vi "add or delete location.vi"(6 "Function":u16(ring) items=["Add/set", "Delete"], 7 "List of defaults":T1 {"List of locations"."Position"."Position Y" format="%#.3f"; "List of locations"."Position"."Position X" format="%#.3f"}, 8 "New location":T3 {"Position"."Position Y" format="%#.3f"; "Position"."Position X" format="%#.3f"}, 9 "Location in":u16, 10 "Device in":u16, 11 "List of devices in":T1 {"List of locations"."Position"."Position Y" format="%#.3f"; "List of locations"."Position"."Position X" format="%#.3f"}) -> (1 "Location out":u16, 2 "Device out":u16, 3 "List of devices out":T1 {"List of locations"."Position"."Position Y" format="%#.3f"; "List of locations"."Position"."Position X" format="%#.3f"})   [LabVIEW 2017]
uses:
  device_list.ctl
  device.ctl
  location.ctl
  <vilib>/Utility/miscctls.llb/LVPointTypeDef.ctl
panel:
  in  "Cancel Button 2":bool
  in  "Delete Button":bool
  in  "Location - delete":u16(ring) caption="Location" items=["Center", "<all>"]
  in  "Device - delete":u16(ring) caption="Device" items=["Layout", "<all>"]
  in  "What to shift?":enum32{"Location", "Device", "All devices"}(radio)
  in  "Location description":string
  in  "Device description":string
  in  "OK Button":bool
  in  "Cancel Button":bool
  in  "Location":u16(ring) items=["Center", "<new location>"]
  in  "Device":u16(ring) items=["Layout", "<new device>"]
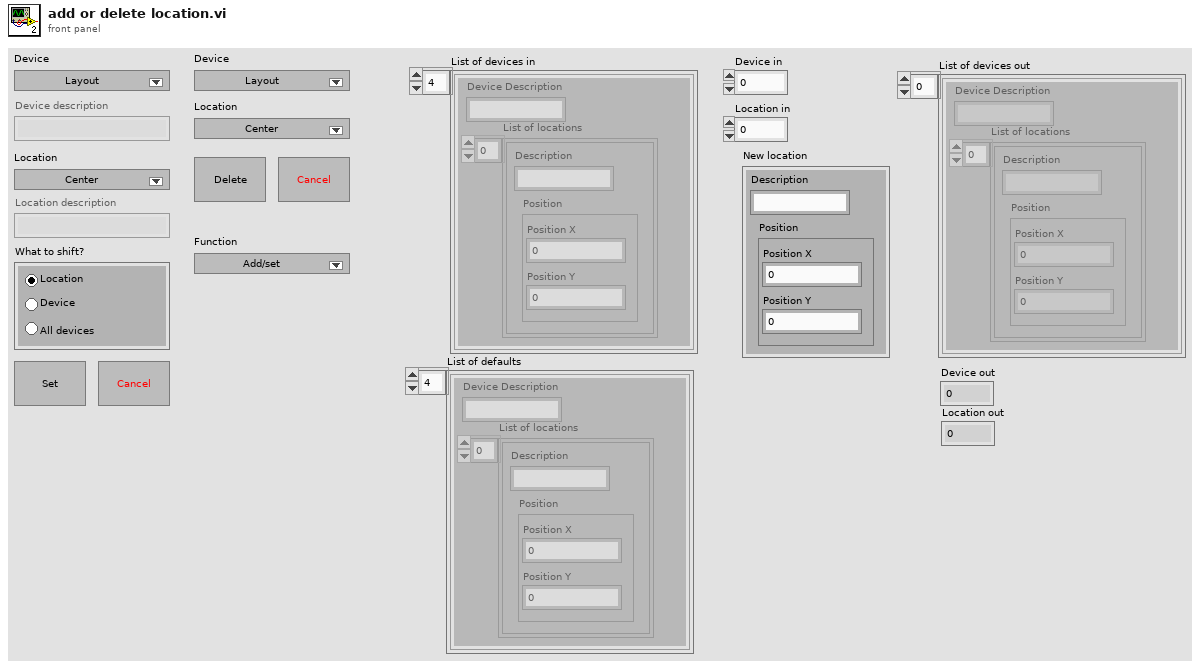
[diagram p1: front panel]
types:
  T1 = typedef "device_list.ctl" = T2[]
  T2 = typedef "device.ctl" = cluster{"List of locations":T3[], "Device Description":string}
  T3 = typedef "location.ctl" = cluster{"Description":string, "Position":cluster{"Position X":dbl, "Position Y":dbl}}
  T4 = typedef "LVRectTypeDef.ctl" = cluster{"Left":i16, "Top":i16, "Right":i16, "Bottom":i16}
  T5 = typedef "LVPointTypeDef.ctl" = cluster{"Horizontal":i16, "Vertical":i16}
  T6 = enum8{"Enabled", "Disabled", "Disabled and Grayed Out"}
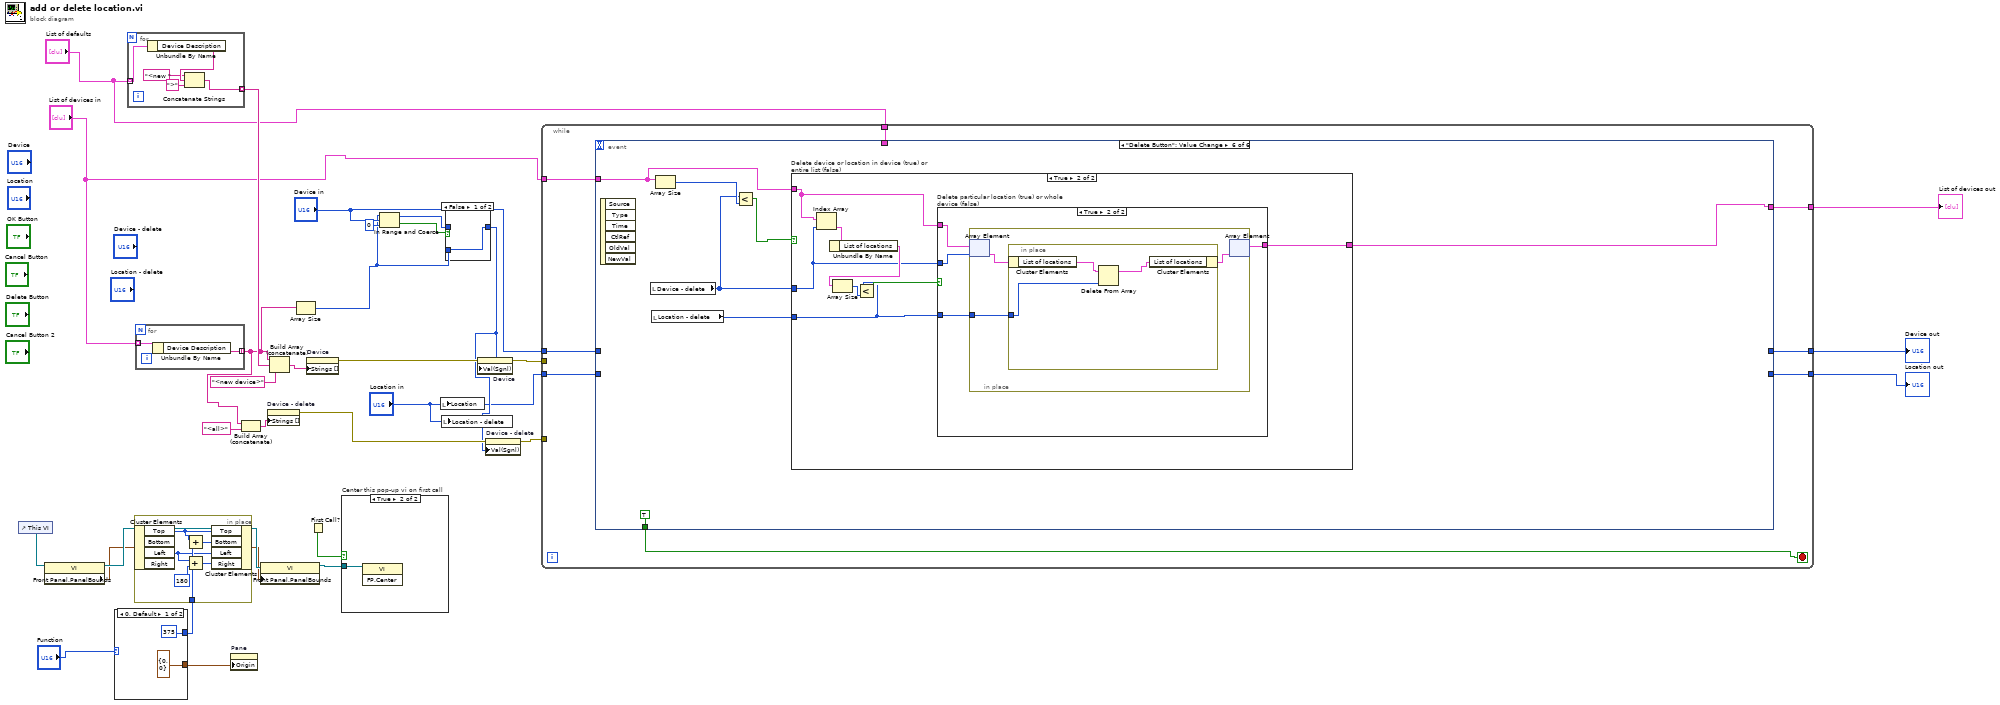
[diagram p0: block diagram]
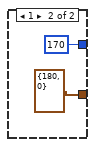
[diagram p2: hidden frame]
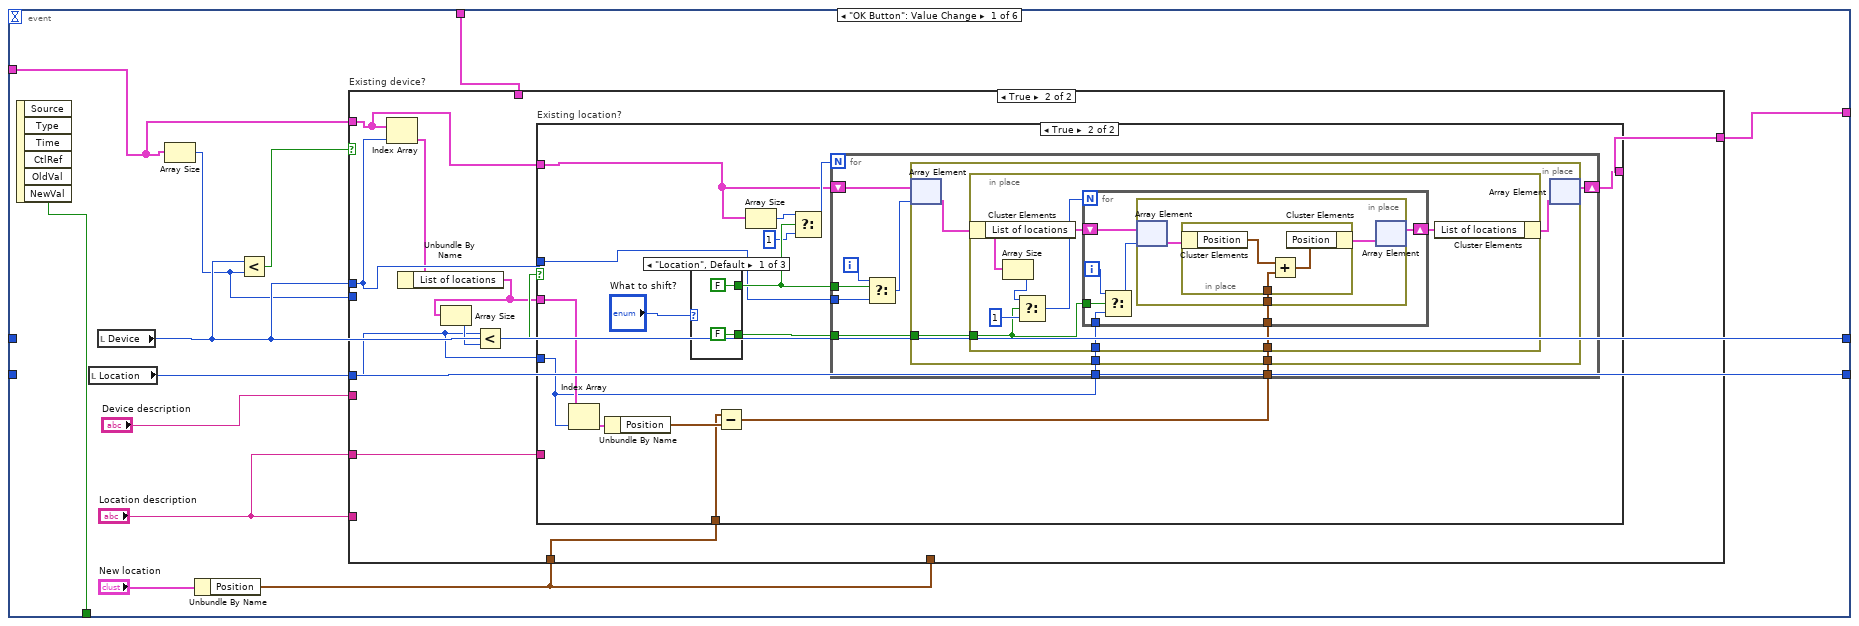
[diagram p5: hidden frame]
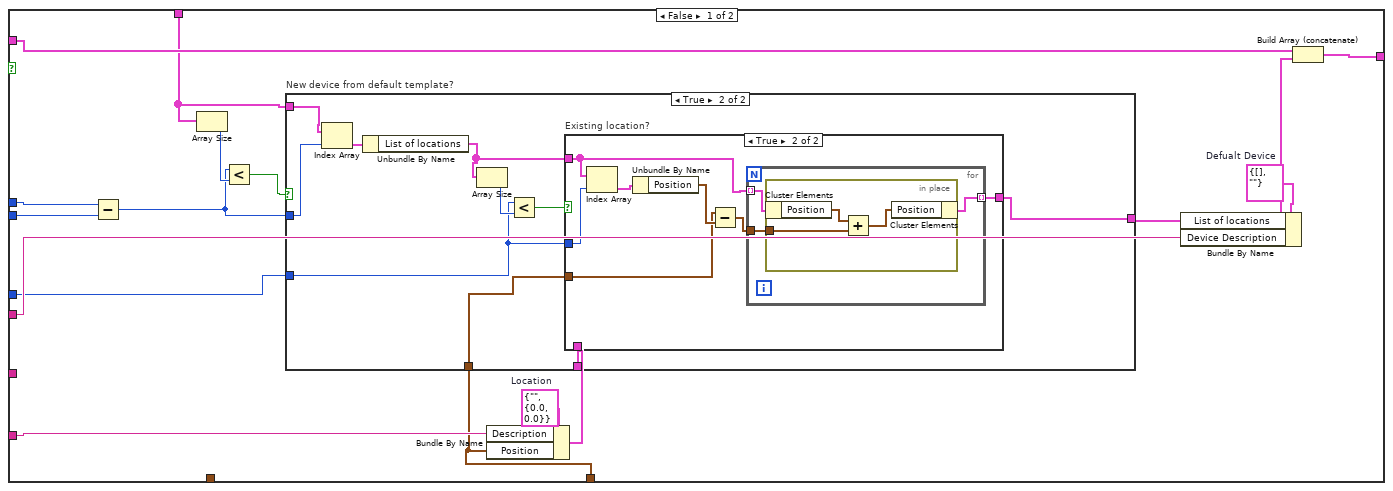
[diagram p6: hidden frame]
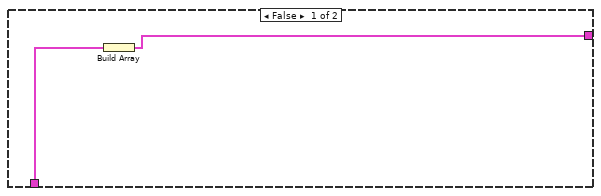
[diagram p7: hidden frame]
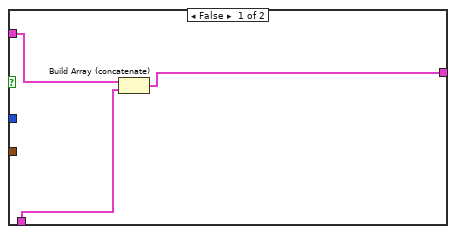
[diagram p8: hidden frame]
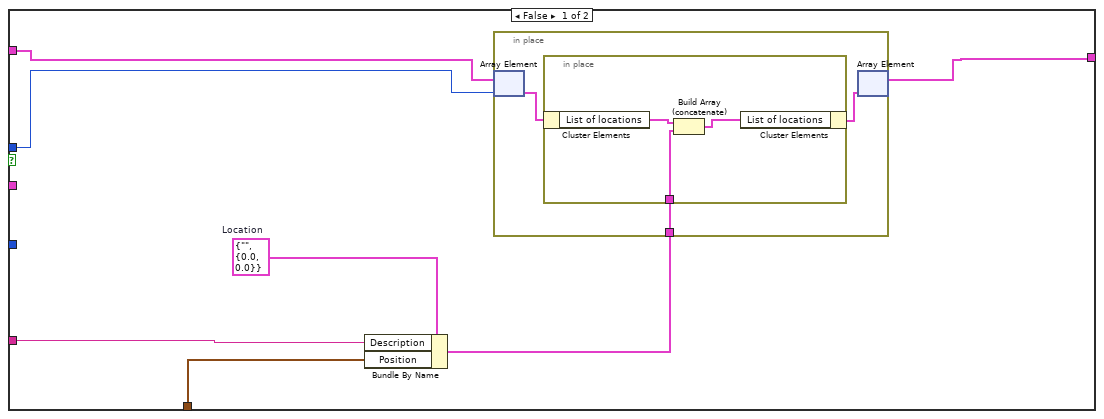
[diagram p9: hidden frame]
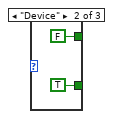
[diagram p10: hidden frame]
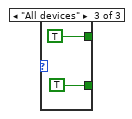
[diagram p11: hidden frame]
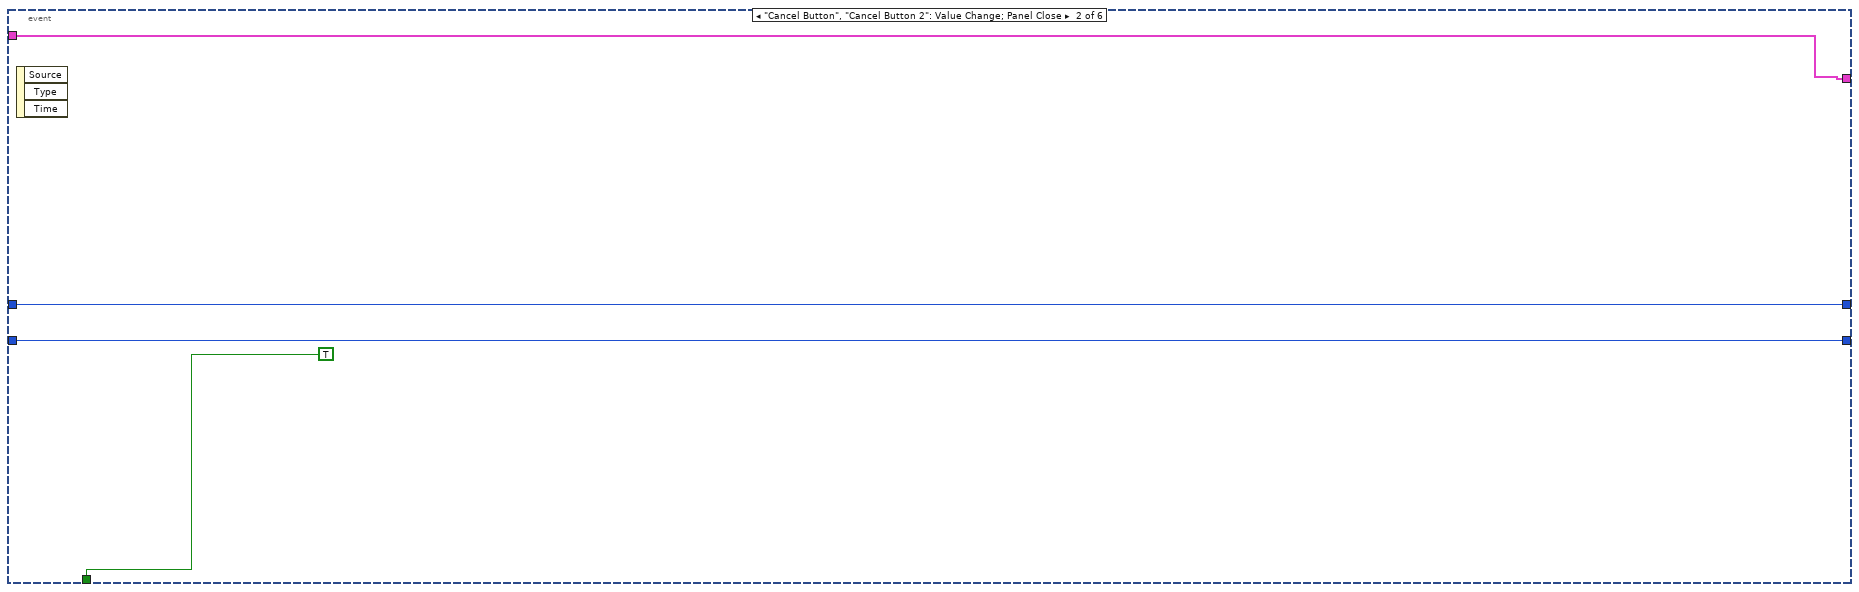
[diagram p12: hidden frame]
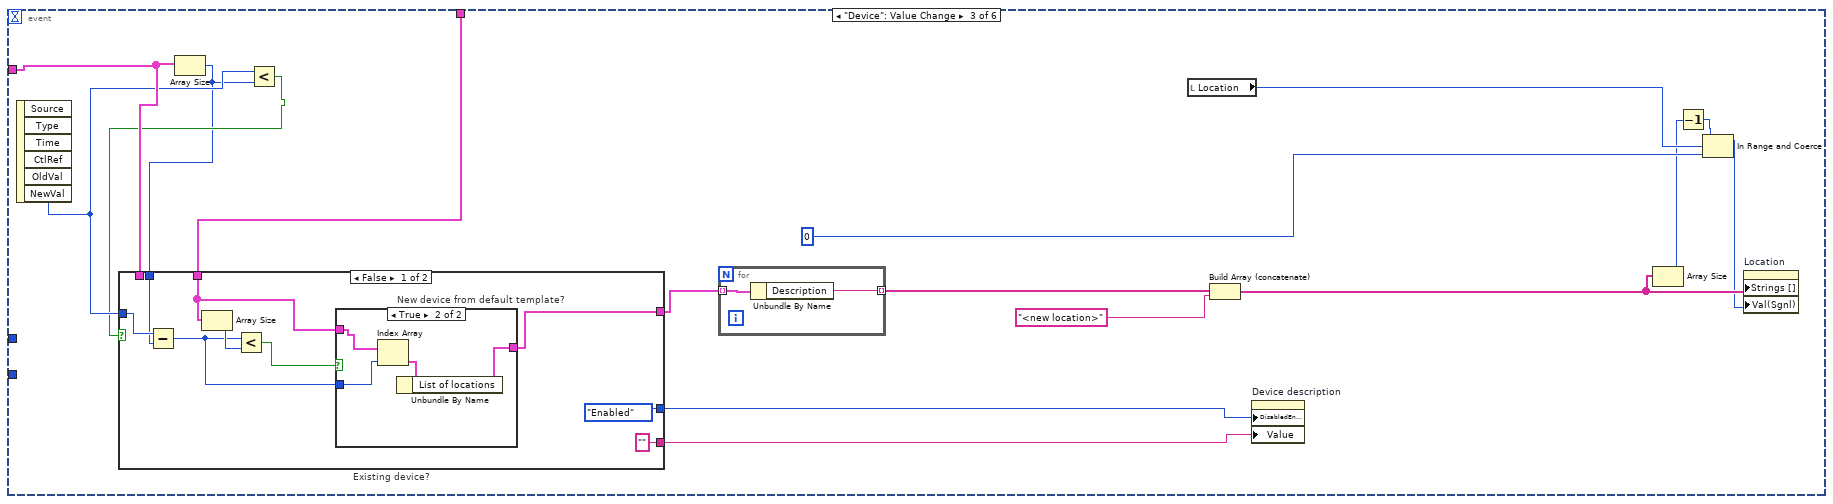
[diagram p13: hidden frame]
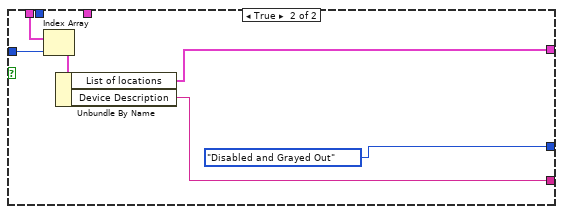
[diagram p15: hidden frame]
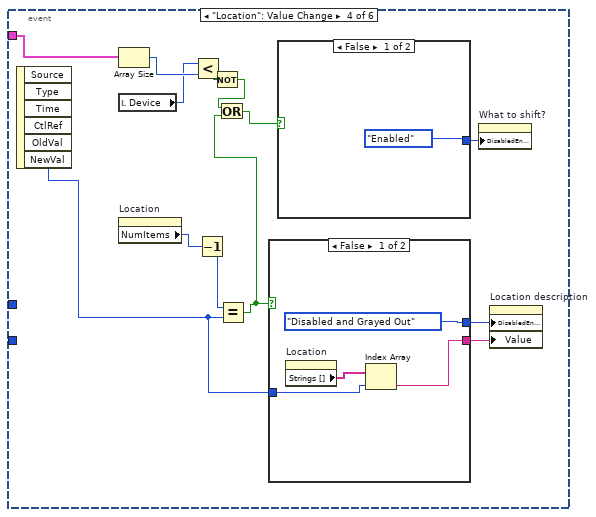
[diagram p16: hidden frame]
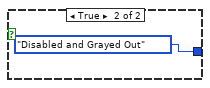
[diagram p17: hidden frame]
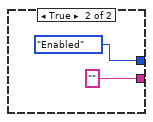
[diagram p18: hidden frame]
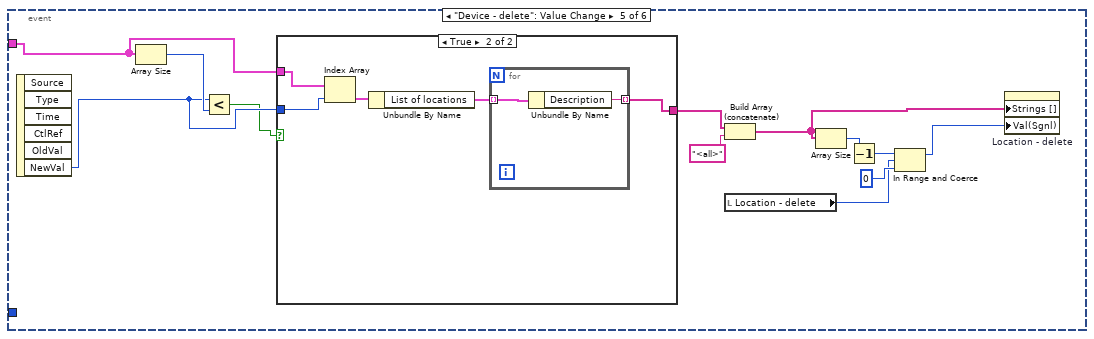
[diagram p19: hidden frame]
diagram:
  n1 = control-ref of="This VI"() -> (w6:refnum<vi>)
  n2 = property class="VI"(reference=w6) -> (reference out=w5:refnum<vi>, "Front Panel.PanelBounds"=w2:T4)  [unwired: 1 in, 1 out]
  n3 = case shown="0, Default" "Function" {
    tunnel: [T5 {"Horizontal"=0, "Vertical"=0} ("Origin") T5 {"Horizontal"=180, "Vertical"=0} ("Origin")] -> w8
    tunnel: [i16 375 ("Horizontal") i16 170 ("Horizontal")] -> w1
    frame 0, Default {
    }
    frame 1 {
    }
  }
  n4 = for {
    tunnel: "List of defaults" -> [w40] mode=indexing
    tunnel: [w36] -> w25 mode=indexing
    n5 = Unbundle By Name(w40) -> ("Device Description"=w39:string)
    n6 = Concatenate Strings("<new " ("string"), w39, ">" ("string")) -> (w36:string)
  }
  n7 = in-place {
    in-place-border: w1 -> [w42]
    n8 = in-place-cluster #1(w2) -> ("Top"=w46:i16, "Left"=w41:i16)  [unwired: 2 out]
    n9 = Add(x=w41, y=i16 180) -> (x+y=w43:i16)
    n10 = Add(x=w46, y=w42) -> (x+y=w45:i16)
    n11 = in-place-cluster #1("Top"=w46, "Bottom"=w45, "Left"=w41, "Right"=w43) -> (w4:T4)
  }
  n12 = for {
    tunnel: "List of devices in" -> [w48] mode=indexing
    tunnel: [w47] -> w19 mode=indexing
    n13 = Unbundle By Name(w48) -> ("Device Description"=w47:string)
  }
  n14 = property on="Pane" class="Pane"("Origin"=w8) -> ()  [unwired: 2 in, 2 out]
  n15 = Build Array (concatenate)(w19, "<all>" ("Device Description")) -> (w17:string[])
  n16 = property class="VI"(reference=w5, "Front Panel.PanelBounds"=w4) -> (reference out=w3:refnum<vi>)  [unwired: 1 in, 1 out]
  n17 = property on="Device - delete" class="Ring (strict)"("Strings []"=w17) -> (error out=w16:errorcluster)  [unwired: 2 in, 1 out]
  n18 = Build Array (concatenate)(w19, w25, "<new device>" ("Device Description")) -> (w24:string[])
  n19 = Array Size(array=w19) -> (size(s)=w13:i32)
  n20 = property on="Device" class="Ring (strict)"("Strings []"=w24) -> (error out=w28:errorcluster)  [unwired: 2 in, 1 out]
  n21 = First Call?() -> (First Call?: T/F=w20:bool)
  n22 = case "Center this pop-up vi on first call" shown="True" w20 {
    tunnel: w3 -> [_ w49]
    frame False {
    }
    frame True {
      n23 = invoke class="VI" method="FP.Center"(reference=w49) -> ()  [unwired: 2 in, 3 out]
    }
  }
  n24 = In Range and Coerce(upper limit=w13, x="Device in", lower limit=0) -> (coerced(x)=w12:i32, In Range?=w11:bool)
  n25 = local write "Location"("Location in") -> ()
  n26 = local write "Location - delete"("Location in") -> ()
  n27 = case shown="False" w11 {
    tunnel: w12 -> [_ w51]
    tunnel: [w50 w51] -> w10
    tunnel: w13 -> [w50 _]
    frame False {
    }
    frame True {
    }
  }
  n28 = property on="Device" class="Ring (strict)"(error in=w28, "Val(Sgnl)"=w10) -> (error out=w27:errorcluster)  [unwired: 1 in, 1 out]
  n29 = property on="Device - delete" class="Ring (strict)"(error in=w16, "Val(Sgnl)"=w10) -> (error out=w15:errorcluster)  [unwired: 1 in, 1 out]
  n30 = while {
    tunnel: "List of devices in" -> [w54]
    tunnel: [w58] -> w31
    tunnel: [w59] -> w26
    tunnel: [w57] -> w30
    tunnel: "Device in" -> [w56]
    tunnel: "Location in" -> [w55]
    tunnel: w27 -> [_]
    tunnel: "List of defaults" -> [w52]
    tunnel: w15 -> [_]
    stop <- w53 stop-if-true
    n31 = event shown="[5] \"Delete Button\": Value Change" {
      selector: _ -> [_ _ _ _ _ _]
      dyn-events: _ -> [_ _ _ _ _ _]
      timeout: _ -> [_ _ _ _ _ _]
      tunnel: w54 -> [w69 w198 w207 w243 w268 w279]
      tunnel: [w66 w198 _ _ _ w278] -> w59
      tunnel: [w71 TRUE ("NewVal") _ _ _ TRUE ("NewVal")] -> w53
      tunnel: [w68 w197 _ _ _ _] -> w58
      tunnel: [w67 w196 _ _ _ _] -> w57
      tunnel: w56 -> [_ w197 _ _ _ _]
      tunnel: w55 -> [_ w196 _ _ _ _]
      tunnel: w52 -> [w62 _ w203 _ _ _]
      event "OK Button": Value Change {
        n32 = event-data() -> ("NewVal"=w71:bool)  [unwired: 1 in, 5 out]
        n33 = local read "Location"() -> (w67:u16)
        n34 = local read "Device"() -> (w68:u16)
        n35 = Array Size(array=w69) -> (size(s)=w63:i32)
        n36 = Unbundle By Name("New location") -> ("Position"=w60:cluster{"Position X":dbl, "Position Y":dbl})
        n37 = Less?(x=w68, y=w63) -> (x < y?=w70:bool)
        n38 = case "Existing device?" shown="True" w70 {
          tunnel: w69 -> [w87 w122]
          tunnel: w68 -> [w83 w121]
          tunnel: w67 -> [w77 w123]
          tunnel: [w85 w119] -> w66
          tunnel: "Location description" -> [_ w124]
          tunnel: "Device description" -> [w84 _]
          tunnel: w60 -> [_ w118]
          tunnel: w63 -> [w82 _]
          tunnel: w62 -> [w78 _]
          tunnel: "Location description" -> [w76 _]
          tunnel: w60 -> [w72 _]
          frame False {
            w74 = T3 {"Description"="", "Position"={"Position X"=0.0, "Position Y"=0.0}}  # Location
            w88 = T2 {"List of locations"=[], "Device Description"=""}  # Defualt Device
            n39 = Subtract(x=w83, y=w82) -> (x-y=w79:i32)
            n40 = Array Size(array=w78) -> (size(s)=w81:i32)
            n41 = Less?(x=w79, y=w81) -> (x < y?=w80:bool)
            n42 = Bundle By Name(cluster=w74, "Description"=w76, "Position"=w72) -> (w73:T3)
            n43 = case "New device from default template?" shown="True" w80 {
              tunnel: w79 -> [_ w99]
              tunnel: w78 -> [_ w100]
              tunnel: w77 -> [_ w94]
              tunnel: [w90 w91] -> w75
              tunnel: w73 -> [w89 w92]
              tunnel: w72 -> [_ w93]
              frame False {
                n44 = Build Array(w89) -> (w90:T3[])
              }
              frame True {
                n45 = Index Array(array=w100, index=w99) -> (element=w98:T2)
                n46 = Unbundle By Name(w98) -> ("List of locations"=w95:T3[])
                n47 = Array Size(array=w95) -> (size(s)=w97:i32)
                n48 = Less?(x=w94, y=w97) -> (x < y?=w96:bool)
                n49 = case "Existing location?" shown="True" w96 {
                  tunnel: w95 -> [w103 w106]
                  tunnel: w94 -> [_ w110]
                  tunnel: w93 -> [_ w107]
                  tunnel: [w101 w105] -> w91
                  tunnel: w92 -> [w102 _]
                  frame False {
                    n50 = Build Array (concatenate)(w103, w102) -> (w101:T3[])
                  }
                  frame True {
                    n51 = Index Array(array=w106, index=w110) -> (element=w109:T3)
                    n52 = Unbundle By Name(w109) -> ("Position"=w108:cluster{"Position X":dbl, "Position Y":dbl})
                    n53 = Subtract(x=w107, y=w108) -> (x-y=w104:cluster{"Position X":dbl, "Position Y":dbl})
                    n54 = for {
                      tunnel: w106 -> [w113] mode=indexing
                      tunnel: [w112] -> w105 mode=indexing
                      tunnel: w104 -> [w111]
                      n55 = in-place {
                        in-place-border: w111 -> [w115]
                        n56 = in-place-cluster #2(w113) -> ("Position"=w116:cluster{"Position X":dbl, "Position Y":dbl})
                        n57 = Add(x=w116, y=w115) -> (x+y=w114:cluster{"Position X":dbl, "Position Y":dbl})
                        n58 = in-place-cluster #2("Position"=w114) -> (w112:T3)
                      }
                    }
                  }
                }
              }
            }
            n59 = Bundle By Name(cluster=w88, "List of locations"=w75, "Device Description"=w84) -> (w86:T2)
            n60 = Build Array (concatenate)(w87, w86) -> (w85:T1)
          }
          frame True {
            n61 = Index Array(array=w122, index=w121) -> (element=w120:T2)
            n62 = Unbundle By Name(w120) -> ("List of locations"=w117:T3[])
            n63 = Array Size(array=w117) -> (size(s)=w126:i32)
            n64 = Less?(x=w123, y=w126) -> (x < y?=w125:bool)
            n65 = case "Existing location?" shown="True" w125 {
              tunnel: w124 -> [w133 _]
              tunnel: w117 -> [_ w154]
              tunnel: w123 -> [_ w142]
              tunnel: w122 -> [w131 w144]
              tunnel: w121 -> [w132 w143]
              tunnel: [w129 w140] -> w119
              tunnel: w118 -> [w128 w141]
              frame False {
                w130 = T3 {"Description"="", "Position"={"Position X"=0.0, "Position Y"=0.0}}  # Location
                n66 = Bundle By Name(cluster=w130, "Description"=w133, "Position"=w128) -> (w127:T3)
                n67 = in-place {
                  in-place-border: w127 -> [w135]
                  n68 = in-place-array #3(w131, w132) -> (w136:T2)
                  n69 = in-place {
                    in-place-border: w135 -> [w138]
                    n70 = in-place-cluster #4(w136) -> ("List of locations"=w139:T3[])
                    n71 = Build Array (concatenate)(w139, w138) -> (w137:T3[])
                    n72 = in-place-cluster #4("List of locations"=w137) -> (w134:T2)
                  }
                  n73 = in-place-array #3(w134) -> (w129:T1)  [unwired: 1 out]
                }
              }
              frame True {
                n74 = Index Array(array=w154, index=w142) -> (element=w153:T3)
                n75 = Unbundle By Name(w153) -> ("Position"=w152:cluster{"Position X":dbl, "Position Y":dbl})
                n76 = case shown="\"Location\", Default" "What to shift?" {
                  tunnel: [FALSE FALSE TRUE] -> w149
                  tunnel: [FALSE TRUE TRUE] -> w148
                  frame "Location", Default {
                  }
                  frame "Device" {
                  }
                  frame "All devices" {
                  }
                }
                n77 = Subtract(x=w141, y=w152) -> (x-y=w145:cluster{"Position X":dbl, "Position Y":dbl})
                n78 = Array Size(array=w144) -> (size(s)=w150:i32)
                n79 = Select(t=w150, s=w149, f=1) -> (s? t:f=w151:i32)
                n80 = for {
                  N: w151 -> [_]
                  shift-right: [w168] -> w140
                  shift-left: w144 -> [w169]
                  tunnel: w149 -> [w166]
                  tunnel: w148 -> [w167]
                  tunnel: w145 -> [w163]
                  tunnel: w143 -> [w162]
                  tunnel: w142 -> [w161]
                  i -> [w165]
                  n81 = Select(t=w165, s=w166, f=w162) -> (s? t:f=w164:i32)
                  n82 = in-place {
                    in-place-border: w167 -> [w172]
                    in-place-border: w163 -> [w171]
                    in-place-border: w161 -> [w170]
                    n83 = in-place-array #5(w169, w164) -> (w174:T2)
                    n84 = in-place {
                      in-place-border: w172 -> [w177]
                      in-place-border: w171 -> [w176]
                      in-place-border: w170 -> [w175]
                      n85 = in-place-cluster #6(w174) -> ("List of locations"=w181:T3[])
                      n86 = Array Size(array=w181) -> (size(s)=w180:i32)
                      n87 = Select(t=w180, s=w177, f=1) -> (s? t:f=w179:i32)
                      n88 = for {
                        N: w179 -> [_]
                        shift-right: [w188] -> w182
                        shift-left: w181 -> [w189]
                        tunnel: w177 -> [w186]
                        tunnel: w176 -> [w184]
                        tunnel: w175 -> [w183]
                        i -> [w187]
                        n89 = Select(t=w187, s=w186, f=w183) -> (s? t:f=w185:i32)
                        n90 = in-place {
                          in-place-border: w184 -> [w190]
                          n91 = in-place-array #7(w189, w185) -> (w192:T3)
                          n92 = in-place {
                            in-place-border: w190 -> [w193]
                            n93 = in-place-cluster #8(w192) -> ("Position"=w195:cluster{"Position X":dbl, "Position Y":dbl})
                            n94 = Add(x=w195, y=w193) -> (x+y=w194:cluster{"Position X":dbl, "Position Y":dbl})
                            n95 = in-place-cluster #8("Position"=w194) -> (w191:T3)
                          }
                          n96 = in-place-array #7(w191) -> (w188:T3[])  [unwired: 1 out]
                        }
                      }
                      n97 = in-place-cluster #6("List of locations"=w182) -> (w173:T2)
                    }
                    n98 = in-place-array #5(w173) -> (w168:T1)  [unwired: 1 out]
                  }
                }
              }
            }
          }
        }
      }
      event "Cancel Button", "Cancel Button 2": Value Change; Panel Close {
        n99 = event-data() -> ()  [unwired: 1 in, 3 out]
      }
      event "Device": Value Change {
        n100 = event-data() -> ("NewVal"=w206:u16)  [unwired: 1 in, 5 out]
        n101 = Array Size(array=w207) -> (size(s)=w202:i32)
        n102 = Less?(x=w206, y=w202) -> (x < y?=w205:bool)
        n103 = case "Existing device?" shown="False" w205 {
          tunnel: w206 -> [w223 w235]
          tunnel: w207 -> [_ w236]
          tunnel: [w218 w231] -> w200
          tunnel: [T6."Enabled" ("Disabled") T6."Disabled and Grayed Out" ("Disabled")] -> w208
          tunnel: ["" ("New device description") w232] -> w204
          tunnel: w203 -> [w220 _]
          tunnel: w202 -> [w222 _]
          frame False {
            n104 = Subtract(x=w223, y=w222) -> (x-y=w219:i32)
            n105 = Array Size(array=w220) -> (size(s)=w224:i32)
            n106 = Less?(x=w219, y=w224) -> (x < y?=w221:bool)
            n107 = case "New device from default template?" shown="True" w221 {
              tunnel: w220 -> [_ w230]
              tunnel: w219 -> [_ w229]
              tunnel: [_ w227] -> w218
              frame False {
              }
              frame True {
                n108 = Index Array(array=w230, index=w229) -> (element=w228:T2)
                n109 = Unbundle By Name(w228) -> ("List of locations"=w227:T3[])
              }
            }
          }
          frame True {
            n110 = Index Array(array=w236, index=w235) -> (element=w234:T2)
            n111 = Unbundle By Name(w234) -> ("List of locations"=w231:T3[], "Device Description"=w232:string)
          }
        }
        n112 = for {
          tunnel: w200 -> [w217] mode=indexing
          tunnel: [w216] -> w201 mode=indexing
          n113 = Unbundle By Name(w217) -> ("Description"=w216:string)
        }
        n114 = local read "Location"() -> (w214:u16)
        n115 = Build Array (concatenate)(w201, "<new location>") -> (w212:string[])
        n116 = property on="Device description" class="Str"("DisabledEnum"=w208, "Value"=w204) -> ()  [unwired: 2 in, 2 out]
        n117 = Array Size(array=w212) -> (size(s)=w210:i32)
        n118 = Decrement(x=w210) -> (x-1=w209:i32)
        n119 = In Range and Coerce(upper limit=w209, x=w214, lower limit=0) -> (coerced(x)=w211:i32)  [unwired: 1 out]
        n120 = property on="Location" class="Ring (strict)"("Strings []"=w212, "Val(Sgnl)"=w211) -> ()  [unwired: 2 in, 2 out]
      }
      event "Location": Value Change {
        n121 = event-data() -> ("NewVal"=w245:u16)  [unwired: 1 in, 5 out]
        n122 = Array Size(array=w243) -> (size(s)=w244:i32)
        n123 = local read "Device"() -> (w239:u16)
        n124 = property on="Location" class="Ring (strict)"() -> ("NumItems"=w249:u32)  [unwired: 2 in, 2 out]
        n125 = Less?(x=w239, y=w244) -> (x < y?=w238:bool)
        n126 = Decrement(x=w249) -> (x-1=w248:u32)
        n127 = Not(x=w238) -> (.not. x?=w237:bool)
        n128 = Equal?(x=w248, y=w245) -> (x = y?=w242:bool)
        n129 = Or(x=w237, y=w242) -> (x .or. y?=w241:bool)
        n130 = case shown="False" w242 {
          tunnel: [T6."Disabled and Grayed Out" ("Disabled") T6."Enabled" ("Disabled")] -> w247
          tunnel: [w252 "" ("New location description")] -> w246
          tunnel: w245 -> [w253 _]
          frame False {
            n131 = property on="Location" class="Ring (strict)"() -> ("Strings []"=w254:string[])  [unwired: 2 in, 2 out]
            n132 = Index Array(array=w254, index=w253) -> (element=w252:string)
          }
          frame True {
          }
        }
        n133 = case shown="False" w241 {
          tunnel: [T6."Enabled" ("Disabled") T6."Disabled and Grayed Out" ("Disabled")] -> w240
          frame False {
          }
          frame True {
          }
        }
        n134 = property on="What to shift?" class="RadioBtnsControl (strict)"("DisabledEnum"=w240) -> ()  [unwired: 2 in, 2 out]
        n135 = property on="Location description" class="Str"("DisabledEnum"=w247, "Value"=w246) -> ()  [unwired: 2 in, 2 out]
      }
      event "Device - delete": Value Change {
        n136 = event-data() -> ("NewVal"=w267:u16)  [unwired: 1 in, 5 out]
        n137 = Array Size(array=w268) -> (size(s)=w269:i32)
        n138 = Less?(x=w267, y=w269) -> (x < y?=w266:bool)
        n139 = case shown="True" w266 {
          tunnel: w268 -> [_ w274]
          tunnel: w267 -> [_ w273]
          tunnel: [_ w270] -> w260
          frame False {
          }
          frame True {
            n140 = Index Array(array=w274, index=w273) -> (element=w272:T2)
            n141 = Unbundle By Name(w272) -> ("List of locations"=w271:T3[])
            n142 = for {
              tunnel: w271 -> [w276] mode=indexing
              tunnel: [w275] -> w270 mode=indexing
              n143 = Unbundle By Name(w276) -> ("Description"=w275:string)
            }
          }
        }
        n144 = Build Array (concatenate)(w260, "<all>" ("Description")) -> (w258:string[])
        n145 = local read "Location - delete"() -> (w262:u16)
        n146 = Array Size(array=w258) -> (size(s)=w265:i32)
        n147 = Decrement(x=w265) -> (x-1=w264:i32)
        n148 = In Range and Coerce(upper limit=w264, x=w262, lower limit=0) -> (coerced(x)=w261:i32)  [unwired: 1 out]
        n149 = property on="Location - delete" class="Ring (strict)"("Strings []"=w258, "Val(Sgnl)"=w261) -> ()  [unwired: 2 in, 2 out]
      }
      event "Delete Button": Value Change {
        n150 = event-data() -> ()  [unwired: 1 in, 6 out]
        n151 = local read "Device - delete"() -> (w281:u16)
        n152 = local read "Location - delete"() -> (w280:u16)
        n153 = Array Size(array=w279) -> (size(s)=w283:i32)
        n154 = Less?(x=w281, y=w283) -> (x < y?=w282:bool)
        n155 = case "Delete device or location in device (true) or entire list (false)" shown="True" w282 {
          tunnel: w281 -> [_ w285]
          tunnel: w280 -> [_ w289]
          tunnel: w279 -> [_ w286]
          tunnel: [_ w284] -> w278
          frame False {
          }
          frame True {
            n156 = Index Array(array=w286, index=w285) -> (element=w288:T2)
            n157 = Unbundle By Name(w288) -> ("List of locations"=w287:T3[])
            n158 = Array Size(array=w287) -> (size(s)=w291:i32)
            n159 = Less?(x=w289, y=w291) -> (x < y?=w290:bool)
            n160 = case "Delete particular location (true) or whole device (false)" shown="True" w290 {
              tunnel: w289 -> [_ w296]
              tunnel: w286 -> [w294 w298]
              tunnel: w285 -> [w293 w297]
              tunnel: [w292 w295] -> w284
              frame False {
                n161 = Delete From Array(array=w294, index=w293) -> (array with subset deleted=w292:T1)  [unwired: 1 in, 1 out]
              }
              frame True {
                n162 = in-place {
                  in-place-border: w296 -> [w300]
                  n163 = in-place-array #9(w298, w297) -> (w301:T2)
                  n164 = in-place {
                    in-place-border: w300 -> [w303]
                    n165 = in-place-cluster #10(w301) -> ("List of locations"=w304:T3[])
                    n166 = Delete From Array(array=w304, index=w303) -> (array with subset deleted=w302:T3[])  [unwired: 1 in, 1 out]
                    n167 = in-place-cluster #10("List of locations"=w302) -> (w299:T2)
                  }
                  n168 = in-place-array #9(w299) -> (w295:T1)  [unwired: 1 out]
                }
              }
            }
          }
        }
      }
    }
  }
  "Device out" <- w31
  "Location out" <- w30
  "List of devices out" <- w26
